vi "Create Execution Unit.vi"(8 "error in":errorcluster, 10 "Item Ref":T2=18446744073709551615 format="%.0x", 11 "Execution Unit Factory Implementation in":refnum<class "Execution Unit Factory.lvclass">) -> (0 "error out":errorcluster, 1 "Asynchronous Execution Units":T1[](array[typedef]) {"ReadWrite Channels" format="%.0x"; "Outgoing Channels" format="%.0x"; "Incoming Channels" format="%.0x"}, 2 "Inline Execution Units":T1[](array[typedef]) {"ReadWrite Channels" format="%.0x"; "Outgoing Channels" format="%.0x"; "Incoming Channels" format="%.0x"}, 3 "Execution Unit Factory Implementation out":refnum<class "Execution Unit Factory.lvclass">)   [LabVIEW 2020, in "Ballard MIL-STD-1553 Engine.lvlib" / "Implementation.lvlib" / "Execution Unit Factory.lvclass"]
uses:
  Execution Unit Factory.lvclass
  Execution Unit/Execution Unit.lvclass
  Interfaces/Execution Unit/Execution Unit.lvclass
  <vilib>/NI VeriStand/Custom Device API/Custom Device Item Ref.ctl
  <vilib>/NI VeriStand/Custom Device API/Custom Device API.lvlib
  Interfaces/Controls/Execution Unit Information.ctl
  Interfaces/Interfaces.lvlib
  Rx Execution Unit/Rx Execution Unit.lvclass
  Tx Execution Unit/Tx Execution Unit.lvclass
  Shared/Parameter Definition.ctl
  Shared/Address.ctl
  Shared/Terminal Endpoint.ctl
  Shared/Message Type.ctl
  Shared/Message Definition.ctl
  Shared/Terminal Name and Address.ctl
  Shared/1553 Channel.ctl
  Shared/1553 Channel Handles.ctl
  C:/dev/niveristand-ballard-milStd1553-custom-device/Source/Custom Device Support/Engine/Implementation/Execution Unit/Execution Unit.lvclass
  C:/dev/niveristand-ballard-milStd1553-custom-device/Source/Custom Device Support/Engine/Interfaces/Execution Unit/Execution Unit.lvclass
  C:/dev/niveristand-ballard-milStd1553-custom-device/Source/Custom Device Support/Engine/Implementation/Rx Execution Unit/Rx Execution Unit.lvclass
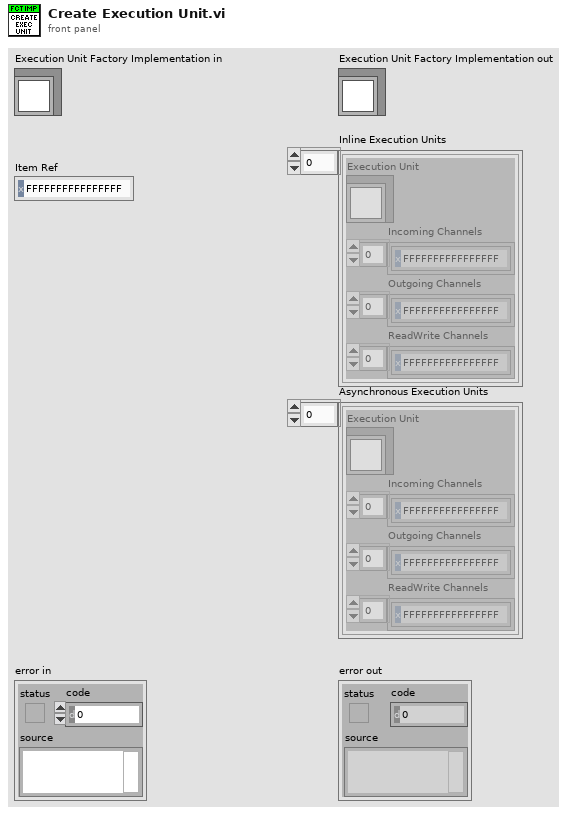
[diagram p1: front panel]
types:
  T1 = typedef "Ballard MIL-STD-1553 Engine.lvlib/Interfaces.lvlib/Execution Unit Information.ctl" = cluster{"Execution Unit":refnum<class "Execution Unit.lvclass">, "Incoming Channels":T2[], "Outgoing Channels":T2[], "ReadWrite Channels":T2[]}
  T2 = typedef "Custom Device API.lvlib/Custom Device Item Ref.ctl" = u64
  T3 = typedef "1553 Channel Handles.ctl" = cluster{"messages":cluster{"parameters":T2[], "timestamps":T2[]}[]}
  T4 = typedef "1553 Channel.ctl" = cluster{"HW channel":u16, "terminals":T5[], "messages":T7[], "acyclic frame names":string[]}
  T5 = typedef "Terminal Name and Address.ctl" = cluster{"name":string, "terminal address":T6}
  T6 = typedef "Address.ctl" = u16
  T7 = typedef "Message Definition.ctl" = cluster{"name":string, "message type":T8, "endpoint Rx":T9, "endpoint Tx":T9, "mode code":u16, "number of words":u16, "parameters":cluster{"name":string, "default value":dbl, "unit":string, "parameter definition":T10}[], "create timestamp channel":bool}
  T8 = typedef "Message Type.ctl" = string
  T9 = typedef "Terminal Endpoint.ctl" = cluster{"terminal address":T6, "subaddress":T6}
  T10 = typedef "Parameter Definition.ctl" = cluster{"start index":i32, "size (bits)":i32, "encoding":enum16{"BNR", "BCD", "Discrete"}, "signed":bool, "multiplier":dbl, "offset":dbl}
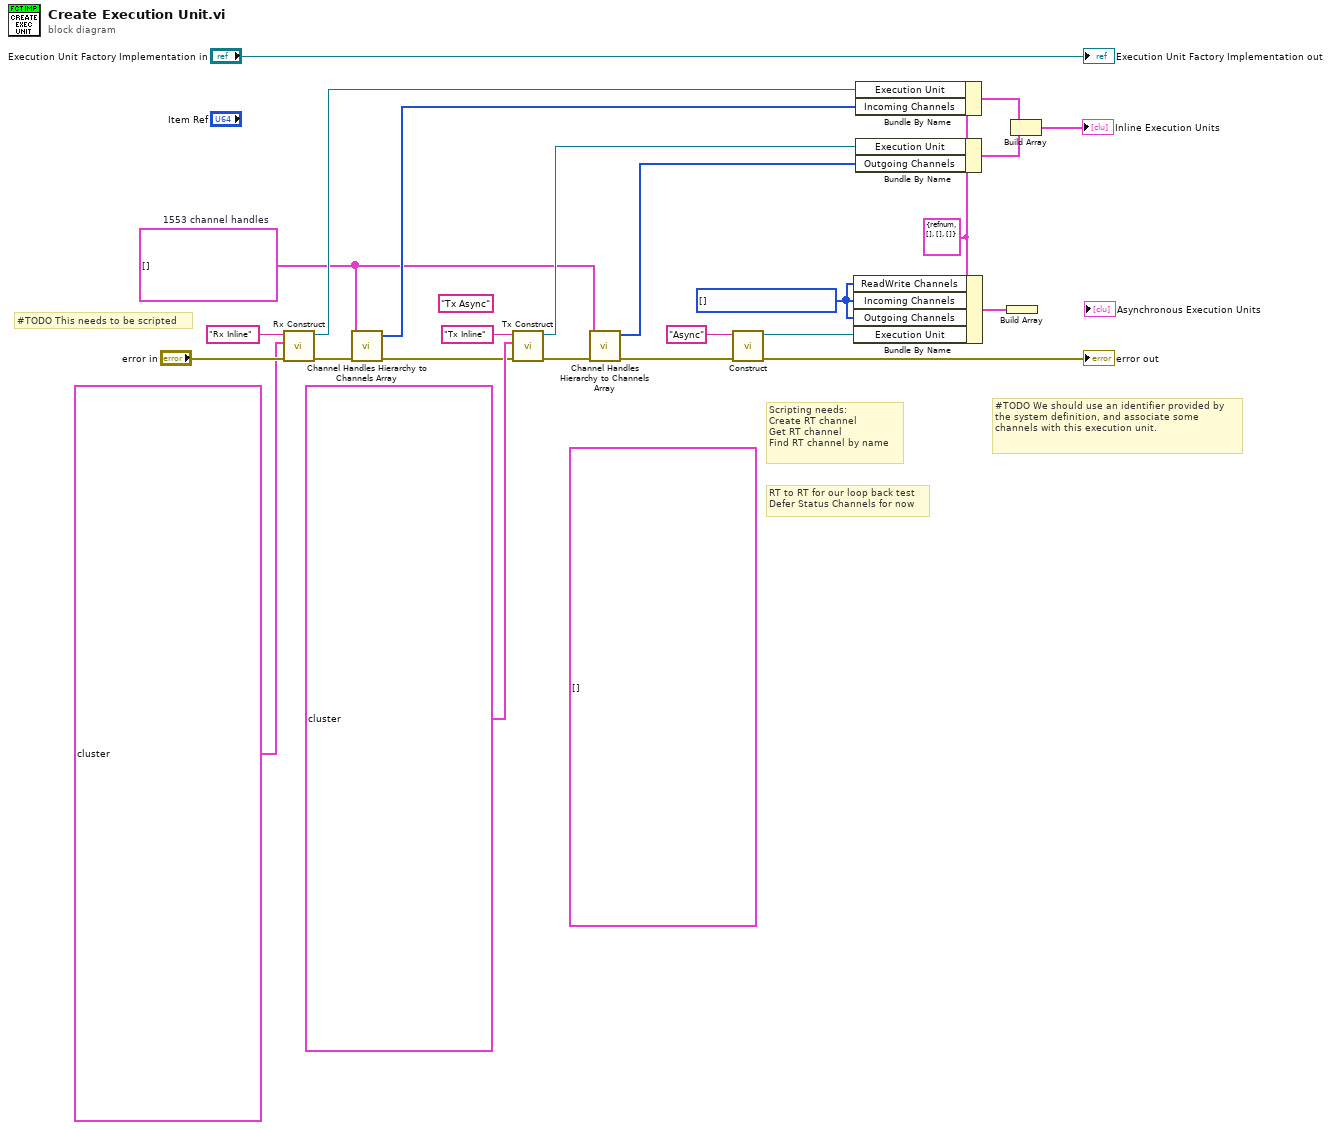
[diagram p0: block diagram]
diagram:
  w1 = T3[] []  # 1553 channel handles
  (unwired) T4[] [] ("1553 channels")
  (unwired) "Tx Async" ("id")
  w22 = T2[] [] ("Incoming Channels")
  w9 = T1 {"Execution Unit"=refnum, "Incoming Channels"=[], "Outgoing Channels"=[], "ReadWrite Channels"=[]} ("Execution Unit Information")
  # "#TODO This needs to be scripted"
  # "Scripting needs:\nCreate RT channel\nGet RT channel\nFind RT channel by name"
  # "RT to RT for our loop back test\nDefer Status Channels for now"
  # "#TODO We should use an identifier provided by the system definition, and associate some channels with this execution unit."
  n1 = call "Rx Construct.vi"("error in"="error in", "1553 channels"=T4[] [{"HW channel"=0, "terminals"=[], "messages"=[{"name"="", "message type"="BC to RT", "endpoint Rx"={"terminal address"=1, "subaddress"=2}, "endpoint Tx"={"terminal address"=0, "subaddress"=0}, "mode code"=0, "number of words"=3, "parameters"=[], "create timestamp channel"=FALSE}, {"name"="", "message type"="RT to RT", "endpoint Rx"={"terminal address"=31, "subaddress"=21}, "endpoint Tx"={"terminal address"=15, "subaddress"=21}, "mode code"=0, "number of words"=11, "parameters"=[], "create timestamp channel"=FALSE}, {"name"="", "message type"="BC to RT", "endpoint Rx"={"terminal address"=1, "subaddress"=3}, "endpoint Tx"={"terminal address"=0, "subaddress"=0}, "mode code"=0, "number of words"=4, "parameters"=[], "create timestamp channel"=FALSE}, {"name"="", "message type"="RT to BC", "endpoint Rx"={"terminal address"=0, "subaddress"=0}, "endpoint Tx"={"terminal address"=1, "subaddress"=5}, "mode code"=0, "number of words"=6, "parameters"=[], "create timestamp channel"=FALSE}, {"name"="", "message type"="RT to BC", "endpoint Rx"={"terminal address"=0, "subaddress"=0}, "endpoint Tx"={"terminal address"=1, "subaddress"=6}, "mode code"=0, "number of words"=2, "parameters"=[], "create timestamp channel"=FALSE}, {"name"="", "message type"="RT to RT", "endpoint Rx"={"terminal address"=15, "subaddress"=20}, "endpoint Tx"={"terminal address"=1, "subaddress"=20}, "mode code"=0, "number of words"=4, "parameters"=[], "create timestamp channel"=FALSE}, {"name"="", "message type"="MC", "endpoint Rx"={"terminal address"=0, "subaddress"=0}, "endpoint Tx"={"terminal address"=1, "subaddress"=31}, "mode code"=16, "number of words"=0, "parameters"=[], "create timestamp channel"=FALSE}, {"name"="", "message type"="MC", "endpoint Rx"={"terminal address"=1, "subaddress"=31}, "endpoint Tx"={"terminal address"=0, "subaddress"=0}, "mode code"=17, "number of words"=0, "parameters"=[], "create timestamp channel"=FALSE}, {"name"="", "message type"="BC to RT", "endpoint Rx"={"terminal address"=31, "subaddress"=28}, "endpoint Tx"={"terminal address"=0, "subaddress"=0}, "mode code"=0, "number of words"=6, "parameters"=[], "create timestamp channel"=FALSE}, {"name"="", "message type"="MC", "endpoint Rx"={"terminal address"=31, "subaddress"=31}, "endpoint Tx"={"terminal address"=0, "subaddress"=0}, "mode code"=1, "number of words"=0, "parameters"=[], "create timestamp channel"=FALSE}], "acyclic frame names"=[]}], "id"="Rx Inline") -> ("error out"=w13:errorcluster, "Rx Execution Unit Implementation out"=w7:refnum<class "Rx Execution Unit.lvclass">)  [unwired: 7 in]
  n2 = call "Channel Handles Hierarchy to Channels Array.vi"("error in"=w13, "1553 channel handles"=w1) -> ("error out"=w12:errorcluster, "Channels"=w6:T2[])  [unwired: 8 in]
  n3 = call "Tx Construct.vi"("error in"=w12, "1553 channels"=T4[] [{"HW channel"=0, "terminals"=[{"name"="TA15", "terminal address"=15}, {"name"="TA31", "terminal address"=31}], "messages"=[{"name"="TA15 to TA31", "message type"="RT to RT", "endpoint Rx"={"terminal address"=31, "subaddress"=21}, "endpoint Tx"={"terminal address"=15, "subaddress"=21}, "mode code"=0, "number of words"=11, "parameters"=[], "create timestamp channel"=FALSE}, {"name"="", "message type"="RT to BC", "endpoint Rx"={"terminal address"=0, "subaddress"=0}, "endpoint Tx"={"terminal address"=1, "subaddress"=5}, "mode code"=0, "number of words"=6, "parameters"=[], "create timestamp channel"=FALSE}, {"name"="", "message type"="BC to RT", "endpoint Rx"={"terminal address"=1, "subaddress"=2}, "endpoint Tx"={"terminal address"=0, "subaddress"=0}, "mode code"=0, "number of words"=3, "parameters"=[], "create timestamp channel"=FALSE}], "acyclic frame names"=[]}], "id"="Tx Inline") -> ("error out"=w5:errorcluster, "Tx Execution Unit Implementation out"=w3:refnum<class "Tx Execution Unit.lvclass">)  [unwired: 7 in]
  n4 = call "Channel Handles Hierarchy to Channels Array.vi"("error in"=w5, "1553 channel handles"=w1) -> ("error out"=w4:errorcluster, "Channels"=w2:T2[])  [unwired: 8 in]
  n5 = call "Construct.vi"("error in (no error)"=w4, "id"="Async") -> ("error out"=→"error out":errorcluster, "Execution Unit Implementation"=w17:refnum<class "Execution Unit.lvclass">)  [unwired: 8 in]
  n6 = Bundle By Name(cluster=w9, "ReadWrite Channels"=w22, "Incoming Channels"=w22, "Outgoing Channels"=w22, "Execution Unit"=w17) -> (w23:T1)
  n7 = Bundle By Name(cluster=w9, "Execution Unit"=w7, "Incoming Channels"=w6) -> (w11:T1)
  n8 = Bundle By Name(cluster=w9, "Execution Unit"=w3, "Outgoing Channels"=w2) -> (w10:T1)
  n9 = Build Array(w23) -> ()  [unwired: 1 out]
  n10 = Build Array(w11, w10) -> (→"Inline Execution Units":T1[])
  "Execution Unit Factory Implementation out" <- "Execution Unit Factory Implementation in"
